vi "REPORT_AUDIT_mark_result.vi"(11 "results_input":string[](array[string])) -> (2 "REPORT_GEAR_statuses":T1, 3 "results_output 2":string[](array[string]))   [LabVIEW 2020]
uses:
  GEAR/typedef/REPORT_GEAR_statuses.ctl
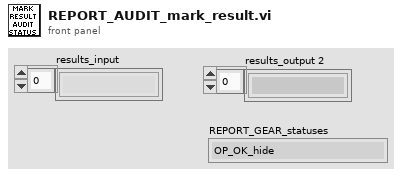
[diagram p1: front panel]
types:
  T1 = typedef "REPORT_GEAR_statuses.ctl" = enum16{"OP_OK_hide", "OP_OK_show", "OP_NOK_hide", "OP_NOK_show", "OP_interrupted_hide", "OP_interrupted_show", "OP_in_operation_hide", "OP_in_operation_show", "OP_unexpected_hide", "OP_unexpected_show", "RE_REAL_OK", "RE_REAL_NOK", "RE_STRING", "RE_sub_header", "RE_no_data", "RE_unexpected", "BA_sub_header", "BA_data", "BA_no_data", "AUDIT_RESULT_OK", "AUDIT_RESULT_NOK", "AUDIT_RESULT_UNEXPECTED"}
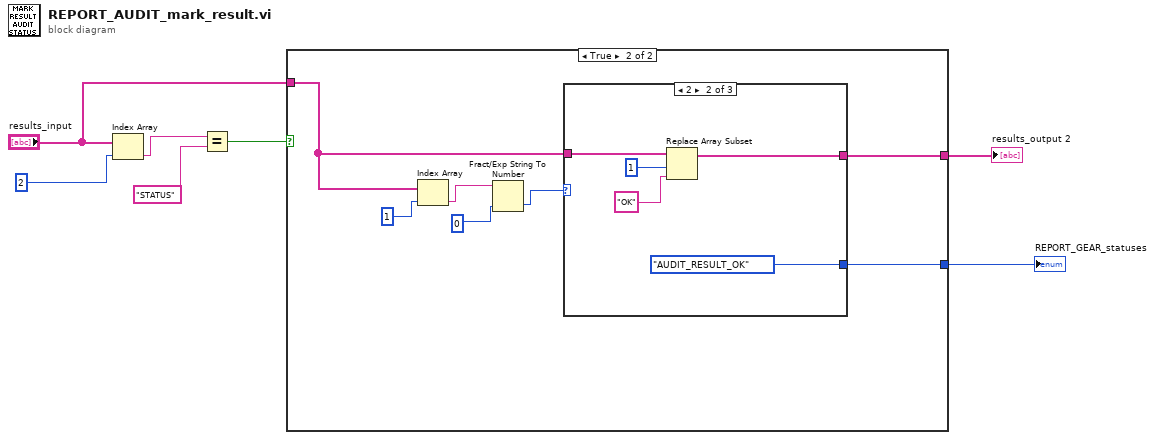
[diagram p0: block diagram]
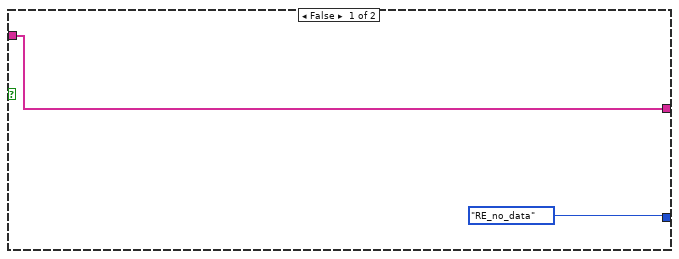
[diagram p2: hidden frame]
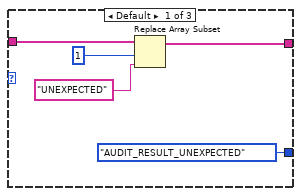
[diagram p3: hidden frame]
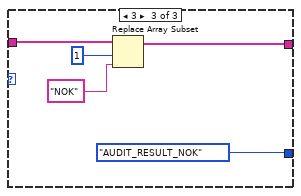
[diagram p4: hidden frame]
diagram:
  n1 = Index Array(array="results_input", index=2) -> (element=w6:string)
  n2 = Equal?(x=w6, y="STATUS") -> (x = y?=w4:bool)
  n3 = case shown="True" w4 {
    tunnel: "results_input" -> [w9 w12]
    tunnel: [REPORT_GEAR_statuses."RE_no_data" ("REPORT_GEAR_statuses") w13] -> w2
    tunnel: [w9 w11] -> w1
    frame False {
    }
    frame True {
      n4 = Index Array(array=w12, index=1) -> (element=w15:string)
      n5 = Fract/Exp String To Number(string=w15, default (0 dbl)=0) -> (number=w10:i32)  [unwired: 2 in, 1 out]
      n6 = case shown="2" w10 {
        tunnel: [REPORT_GEAR_statuses."AUDIT_RESULT_UNEXPECTED" ("REPORT_GEAR_statuses") REPORT_GEAR_statuses."AUDIT_RESULT_OK" ("REPORT_GEAR_statuses") REPORT_GEAR_statuses."AUDIT_RESULT_NOK" ("REPORT_GEAR_statuses")] -> w13
        tunnel: w12 -> [w19 w25 w29]
        tunnel: [w18 w22 w28] -> w11
        frame Default {
          n7 = Replace Array Subset(array=w19, new element="UNEXPECTED", index=1) -> (w18:string[])
        }
        frame 2 {
          n8 = Replace Array Subset(array=w25, new element="OK", index=1) -> (w22:string[])
        }
        frame 3 {
          n9 = Replace Array Subset(array=w29, new element="NOK", index=1) -> (w28:string[])
        }
      }
    }
  }
  "REPORT_GEAR_statuses" <- w2
  "results_output 2" <- w1
